vi "Write Subpanel Name.vi"(2 "error in (no error)":errorcluster, 3 "Name":string, 4 "Controller in":refnum<class "Generic Plugin.lvclass">) -> (0 "error out":errorcluster, 1 "Controller out":refnum<class "Generic Plugin.lvclass">)   [LabVIEW 2020, in "RxnRover.lvlib" / "Generic Plugin.lvclass"]
uses:
  Generic Plugin.lvclass
  Generic Plugin.lvclass/Generic Plugin.ctl
  Sub VIs/Message Queue/Enqueue Message (Single).vi
  Sub VIs/Message Queue/test Message Queue.lvlib
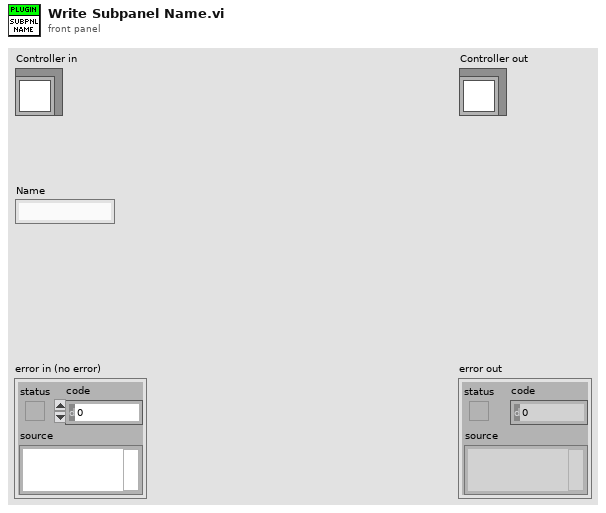
[diagram p1: front panel]
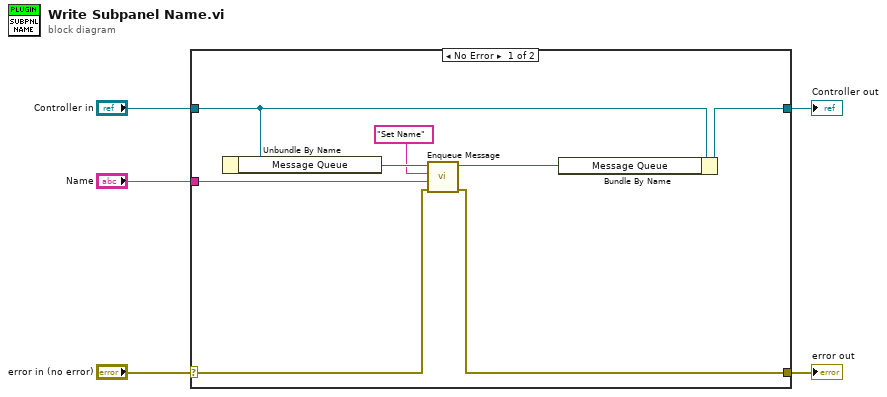
[diagram p0: block diagram]
diagram:
  n1 = case shown="No Error" "error in (no error)" {
    selector: "error in (no error)" -> [w8 w15]
    tunnel: [w7 w15] -> w4
    tunnel: [w10 w14] -> w2
    tunnel: "Controller in" -> [w13 w14]
    tunnel: "Name" -> [w6 _]
    frame No Error {
      n2 = Unbundle By Name(w13) -> ("Message Queue"=w12:refnum<queue>)
      n3 = call-poly "Enqueue Message.vi"("error in (no error)"=w8, "Message Data"=w6, "Message"="Set Name", "Message Queue"=w12) -> ("error out"=w7:errorcluster, "dup Message Queue"=w9:refnum<queue>)  [unwired: 6 in]
      n4 = Bundle By Name(cluster=w13, "Message Queue"=w9) -> (w10:refnum<class "Generic Plugin.lvclass">)
    }
    frame Error {
    }
  }
  "error out" <- w4
  "Controller out" <- w2
